vi "Set All.vi"(9 "Init Value":T1[](array[typedef]), 10 "Previous Value":T1[](array[typedef]), 11 "Set ALL NewVal":bool) -> (3 "Value Out":T1[](array[typedef]))   [LabVIEW 2019, in "Scan Engine Custom Device.lvlib"]
doc: "Set all modules to \"Scan Engine\" mode control (for those supporting it), value changed."
uses:
  Scan Engine Custom Device.lvlib
  Type Defs/Slot Programming Mode.ctl
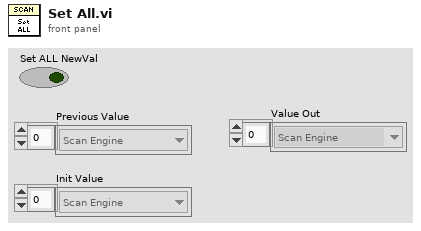
[diagram p1: front panel]
types:
  T1 = typedef "Scan Engine Custom Device.lvlib/Slot Programming Mode.ctl" = enum16{"Scan Engine", "LabVIEW FPGA", "NI-DAQmx", "Don't Modify"}
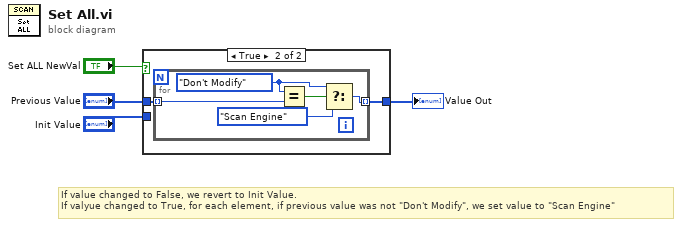
[diagram p0: block diagram]
diagram:
  # "If value changed to False, we revert to Init Value.\nIf valyue changed to True, for each element, if previous value was not \"Don't Modify\", we set value to \"Scan Engine\""
  n1 = case shown="True" "Set ALL NewVal" {
    tunnel: "Previous Value" -> [_ w7]
    tunnel: "Init Value" -> [w5 _]
    tunnel: [w5 w6] -> w4
    frame False {
    }
    frame True {
      n2 = for {
        tunnel: w7 -> [w10] mode=indexing
        tunnel: [w11] -> w6 mode=indexing
        w9 = Slot_Programming_Mode."Don't Modify" ("y")
        n3 = Equal?(x=w9, y=w10) -> (x = y?=w12:bool)
        n4 = Select(t=w9, s=w12, f=Slot_Programming_Mode."Scan Engine") -> (s? t:f=w11:T1)
      }
    }
  }
  "Value Out" <- w4
